vi "Draw Arrowed Line (Greyscale).vi"(4 "Tip Length (Default 0.1)":dbl=0.1, 5 "Thickness (Default: 1)":i32=1, 6 "OpenCV Line Type (Default LINE_8)":T3=enum."LINE_8", 7 "Colour":u8=255, 8 "error in (no error)":errorcluster, 9 "Pointed-to Point":T1, 10 "Start Point":T1, 11 "Greyscale Image":T2) -> (0 "error out":errorcluster, 3 "Greyscale Image (Duplicate)":T2)   [LabVIEW 2020, in "g_ar_toolkit.image.lvlib"]
uses:
  g_ar_toolkit.image.lvlib
  Line Type.ctl
  g_ar_toolkit.common/Image Point (Integer).ctl
  Greyscale Image.ctl
  c990ea83-8feb-41a3-987e-5529af170d73.vi
  g_ar_toolkit.common/Module Path.vi
  <vilib>/Utility/error.llb/Error Cluster From Error Code.vi
  g_ar_toolkit.common/g_ar_toolkit.common.lvlib
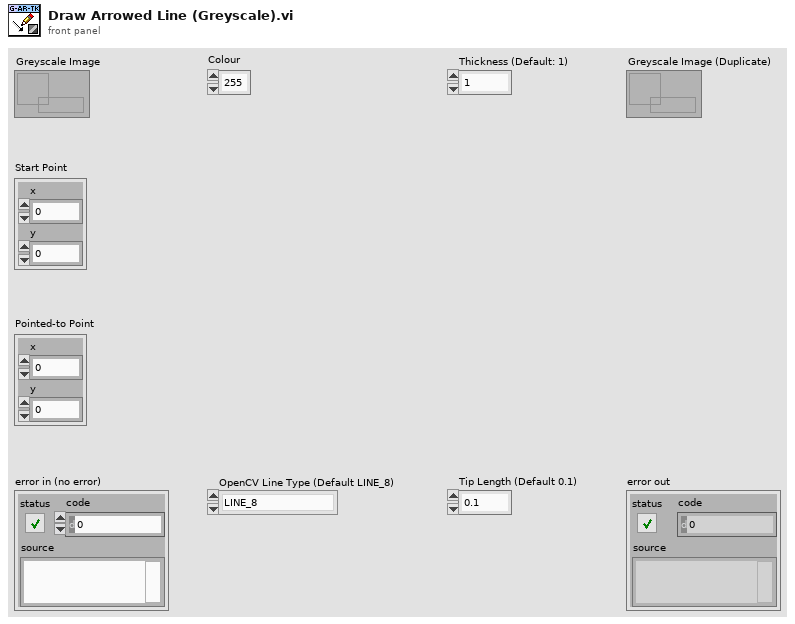
[diagram p1: front panel]
types:
  T1 = typedef "g_ar_toolkit.common.lvlib/Image Point (Integer).ctl" = cluster{"x":i32, "y":i32}
  T2 = typedef "g_ar_toolkit.image.lvlib/Greyscale Image.ctl" = refnum<data-value>
  T3 = typedef "g_ar_toolkit.image.lvlib/Line Type.ctl" = enum8{"FILLED", "LINE_4", "LINE_8", "LINE_AA"}
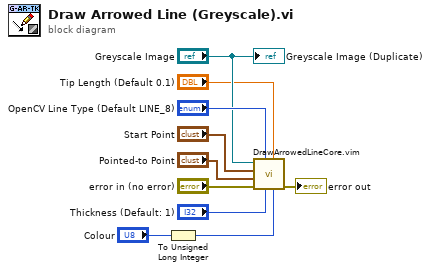
[diagram p0: block diagram]
diagram:
  n1 = To Unsigned Long Integer(number="Colour") -> (unsigned 32bit integer=w4:u32)
  n2 = call "DrawArrowedLineCore.vim"("Colour"=w4, "Tip Length"="Tip Length (Default 0.1)", "Thickness"="Thickness (Default: 1)", "OpenCV Line Type"="OpenCV Line Type (Default LINE_8)", "error in (no error)"="error in (no error)", "Point B"="Pointed-to Point", "Point A"="Start Point", "Src"="Greyscale Image") -> ("error out"=→"error out":errorcluster)  [unwired: 3 in]
  "Greyscale Image (Duplicate)" <- "Greyscale Image"
